vi "RSZVB State Checking.vi"(8 "error in (no error)":errorcluster {"code" format="%.0x"}, 10 "State Checking (T: On)":bool, 11 "VISA session":refnum<visa-resource-name>) -> (0 "error out":errorcluster {"code" format="%.0x"}, 3 "dup VISA session":refnum<visa-resource-name>)   [LabVIEW 2011]
doc: "This VI switches state checking of the instrument (reading of the Standard Event Register and checking it for error) status subsystem. Driver VIs are using state checking which is by default enabled.\n\nNote:\n\n(1) In debug mode enable state checking.\n\n(2) For better bus throughput and instruments performance disable state checking.\n\n(3) When state checking is disabled driver does not check if correct instrument model or option is used with each of the VIs. This might cause unexpected behaviour of the instrument."
uses:
  _utility/RSZVB Global Data.vi
panel:
  # "On\nOff"
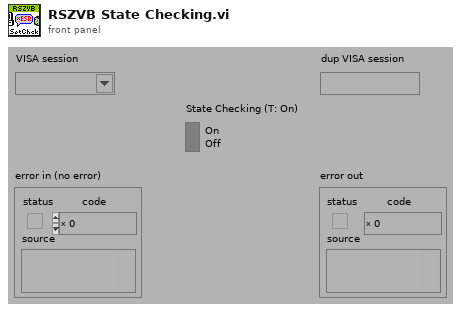
[diagram p1: front panel]
types:
  T1 = cluster{"Error Checking (T: On)":bool, "Installed Options":string[], "Data Valid?":bool, "Ports":i32, "Model":string[], "Option Checking (T: On)":bool}[]
  T2 = cluster{"Error Checking (T: On)":bool, "Installed Options":string[], "Data Valid?":bool, "Ports":i32, "Model":string[], "Option Checking (T: On)":bool}
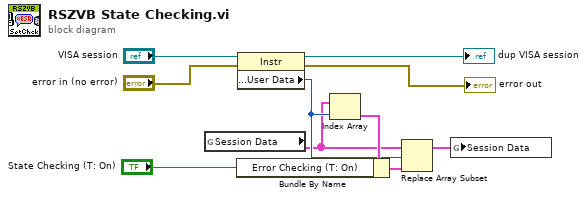
[diagram p0: block diagram]
diagram:
  n1 = global read "RSZVB Global Data.vi" "Session Data"() -> (w6:T1)
  n2 = property class="Instr"(reference="VISA session", error in="error in (no error)") -> (reference out=→"dup VISA session":refnum<visa-resource-name>, error out=→"error out":errorcluster, "General Settings:User Data"=w9:u32)
  n3 = Index Array(array=w6, index=w9) -> (element=w10:T2)
  n4 = Bundle By Name(cluster=w10, "Error Checking (T: On)"="State Checking (T: On)") -> (w8:T2)
  n5 = Replace Array Subset(array=w6, new element=w8, index=w9) -> (w7:T1)
  n6 = global write "RSZVB Global Data.vi" "Session Data"(w7) -> ()
